vi "CheckOutLogic.vi"(10 "Student ID":i32, 11 "all rows":string[][](array[string])) -> (1 "Total Elapsed Time":i32, 2 "Total Seconds Out":string, 3 "Elapsed Seconds":i32)   [LabVIEW 2013]
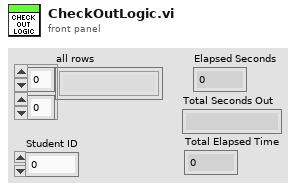
[diagram p1: front panel]
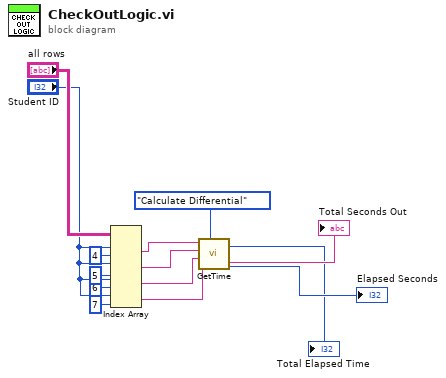
[diagram p0: block diagram]
diagram:
  n1 = Index Array(array="all rows", index (row) #1="Student ID", index (col) #1=4 ("disabled index (col)"), index (row) #2="Student ID", index (col) #2=5 ("disabled index (col)"), index (row) #3="Student ID", index (col) #3=6 ("disabled index (col)"), index (row) #4="Student ID", index (col) #4=7 ("disabled index (col)")) -> (element #1=w9:string, element #2=w10:string, element #3=w11:string, element #4=w5:string)
  n2 = call "GetTime.vi"("State"=enum16{"Get Time", "Calculate Differential"}."Calculate Differential", "Total Seconds"=w5, "Stored Seconds"=w11, "Stored Minutes"=w10, "Stored Hours"=w9) -> ("Elapsed Seconds"=→"Elapsed Seconds":i32, "Total Seconds Out"=→"Total Seconds Out":string, "Total Elapsed Time"=→"Total Elapsed Time":i32)  [unwired: 1 in, 3 out]
